vi "Multiple TransducersNathanOnboardClock.vi"() -> ()   [LabVIEW 2015]
doc: "Reads force and torque values from multiple ATI transducers."
uses:
  <vilib>/DAQmx/read.llb/DAQmx Read (Analog 2D DBL NChan NSamp).vi
  <vilib>/Analysis/baseanly.llb/A x Vector.vi
  <vilib>/DAQmx/create/channels.llb/DAQmx Create Channel (AI-Voltage-Basic).vi
  <vilib>/DAQmx/configure/timing.llb/DAQmx Timing (Sample Clock).vi
  <vilib>/DAQmx/configure/trigger.llb/DAQmx Start Trigger (Digital Edge).vi
  <vilib>/DAQmx/miscellaneous.llb/DAQmx Fill In Error Info.vi
  <vilib>/Analysis/NI_AALBase.lvlib
panel:
  in  "User Torque Units":string
  in  "User Force Units":string
  in  "Calibration Units":T1(array[cluster])
  in  "Tool Transforms":T2(array[cluster])
  in  "Scan Lists":string[](array[string])=["dev1/ai0:5,dev1/ai6:11"]
  in  "Enable Transducer":bool[](array[boolean])
  in  "Filename":path
  in  "Connection Mode":i32(ring)=-1 items=["default"=-1, "RSE"=10083, "NRSE"=10078, "Differential"=10106, "Pseudodifferential"=12529]
  in  "Bias All":bool
  in  "Start Saving Data":bool
  in  "Bias Transducer":bool[](array[boolean])
  in  "Append Data?":bool
  in  "Samples to Read at a time":i32=50
  out "Voltages":dbl[][](array[numeric])
  in  "Buffer Size":i32=1000
  in  "Sample Rate":dbl=1000.0
  out "F/T Values":dbl[][][](array[numeric])
  in  "Calibration Files":path[](array[path])=[path "C:/Program Files/ATI DAQ FT/FT5816.cal", path "C:/Program Files/ATI DAQ FT/FT5395.cal"]
  # "For assistance, turn on context help and examine\nthe help text for each control."
  # "Fx"
  # "Fy"
  # "Fz"
  # "Tx"
  # "Ty"
  # "Tz"
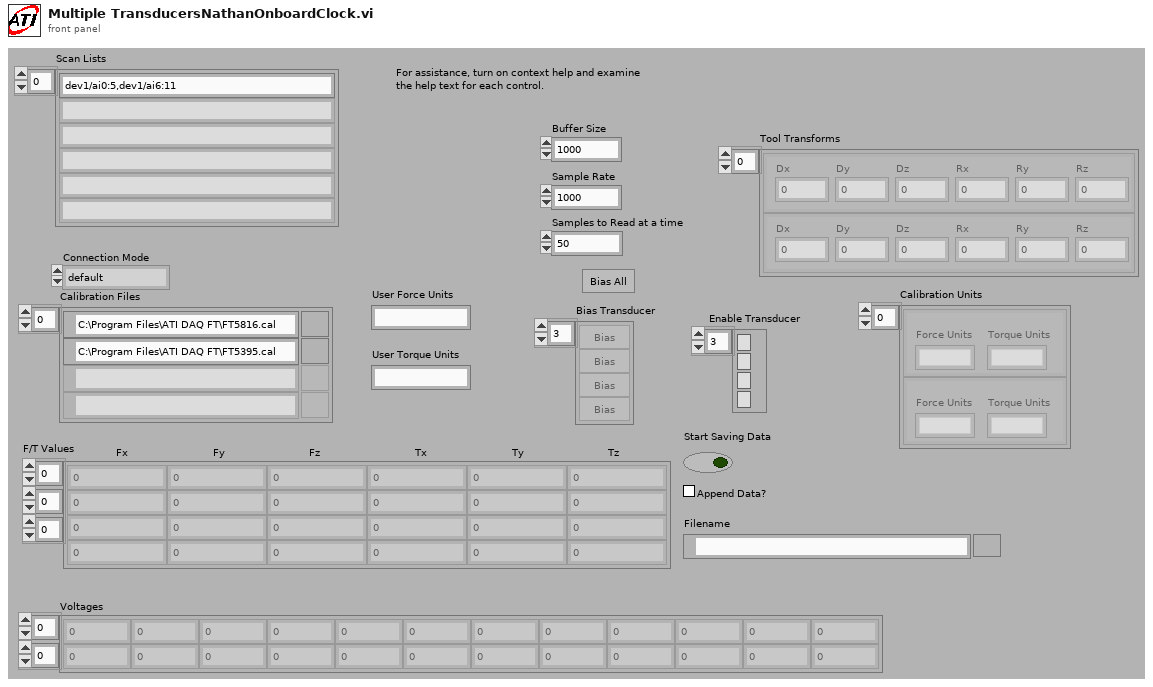
[diagram p1: front panel]
types:
  T1 = cluster{"Force Units":string, "Torque Units":string}[]
  T2 = cluster{"Dx":dbl, "Dy":dbl, "Dz":dbl, "Rx":dbl, "Ry":dbl, "Rz":dbl}[]
  T3 = cluster{"Calibration Force Units":string, "Calibration Torque Units":string}
  T4 = enum16{"open", "open or create", "create or replace", "create", "open (read only)"}
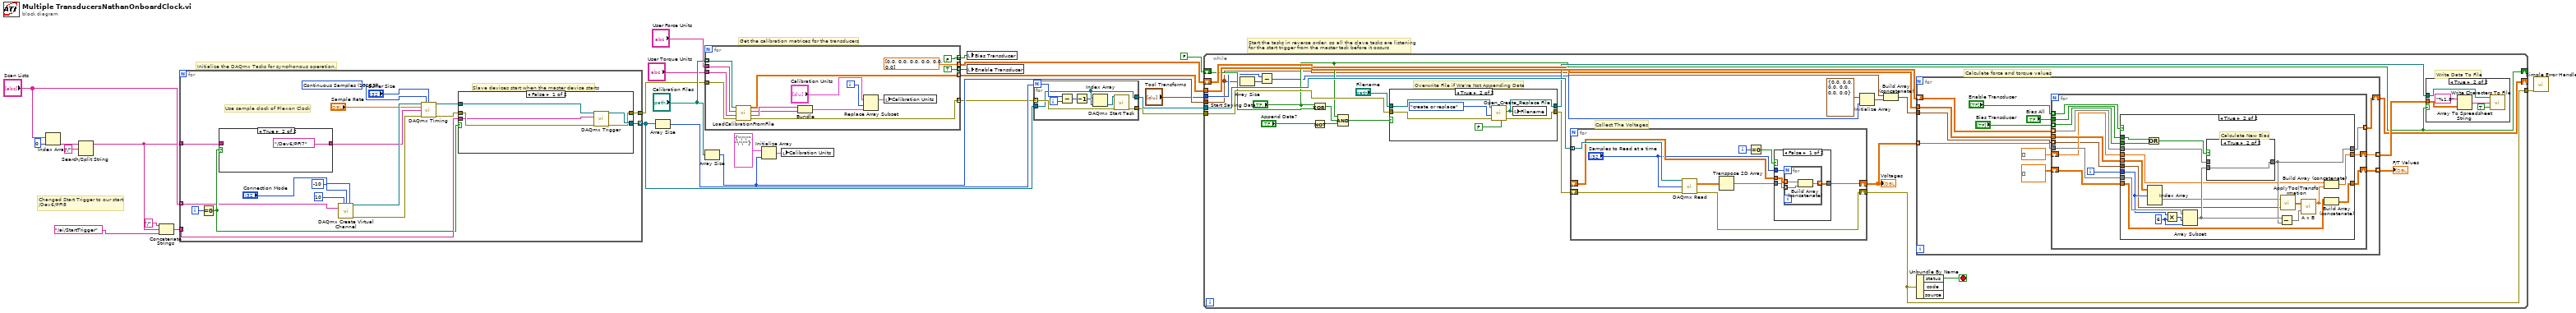
[diagram p0: block diagram]
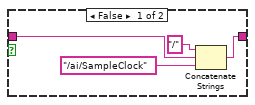
[diagram p7: hidden frame]
diagram:
  # "Changed Start Trigger to our start\n/Dev6/PFI8"
  # "Initialize the DAQmx Tasks for syncrhonous operation."
  # "Get the calibration matrices for the transducers"
  # "Start the tasks in reverse order, so all the slave tasks are listening \nfor the start trigger from the master task before it occurs"
  n1 = Index Array(array="Scan Lists", index=0) -> (element=w15:string)
  n2 = Search/Split String(string=w15, search string/char (-)="/") -> (substring before match=w13:string)  [unwired: 1 in, 2 out]
  n3 = Concatenate Strings("/", w13, "/ai/StartTrigger") -> (w27:string)
  n4 = for {
    tunnel: w27 -> [w39]
    tunnel: [w36] -> w3
    tunnel: [w30] -> w18 mode=indexing
    tunnel: "Scan Lists" -> [w29] mode=indexing
    tunnel: w13 -> [w28]
    i -> [w41]
    w43 = 10123 items=["Finite Samples"=10178, "Continuous Samples"=10123, "Hardware Timed Single Point"=12522] ("sample mode")
    # "Slave devices start when the master device starts"
    # "Use sample clock of Plexon Clock"
    n5 = Equal To 0?(x=w41) -> (x = 0?=w35:bool)
    n6 = case shown="True" w35 {
      tunnel: [w47 tag "/Dev6/PFI7"] -> w34
      tunnel: w28 -> [w46 _]
      frame False {
        n7 = Concatenate Strings("/", w46, "/ai/SampleClock") -> (w47:string)
      }
      frame True {
      }
    }
    n8 = call-poly <vilib>:"DAQmx Create Virtual Channel.vi"("maximum value"=10, "minimum value"=-10, "input terminal configuration"="Connection Mode", "physical channels"=w29) -> ("task out"=w45:refnum<k21>, "error out"=w38:errorcluster)  [unwired: 10 in]
    n9 = call-poly <vilib>:"DAQmx Timing.vi"("task/channels in"=w45, "sample mode"=w43, "samples per channel"="Buffer Size", "rate"="Sample Rate", "source"=w34, "error in"=w38) -> ("task out"=w40:refnum<k21>, "error out"=w37:errorcluster)  [unwired: 8 in]
    n10 = case shown="False" w35 {
      tunnel: w40 -> [w55 w57]
      tunnel: [w54 w57] -> w30
      tunnel: w39 -> [w51 _]
      tunnel: w37 -> [w53 w56]
      tunnel: [w52 w56] -> w36
      frame False {
        n11 = call-poly <vilib>:"DAQmx Trigger.vi"("task/channels in"=w55, "source"=w51, "error in"=w53) -> ("task out"=w54:refnum<k21>, "error out"=w52:errorcluster)  [unwired: 11 in]
      }
      frame True {
      }
    }
  }
  n12 = Array Size(array=w18) -> (size(s)=w20:i32)
  n13 = for {
    tunnel: "Calibration Files" -> [w70] mode=indexing
    tunnel: [FALSE] -> w24 mode=indexing
    tunnel: [TRUE] -> w22 mode=indexing
    tunnel: [w68] -> w21 mode=indexing
    tunnel: [dbl[] [0.0, 0.0, 0.0, 0.0, 0.0, 0.0]] -> w11 mode=indexing
    tunnel: "User Force Units" -> [w61]
    tunnel: "User Torque Units" -> [w60]
    tunnel: w3 -> [w59]
    tunnel: [w58] -> w2 mode=indexing
    i -> [w67]
    n14 = call "LoadCalibrationFromFile.vi"("Error In"=w59, "User Torque Units"=w60, "User Force Units"=w61, "Cal File Path"=w70) -> ("Error Out"=w58:errorcluster, "Calibration Force Units"=w64:string, "Calibration Torque Units"=w63:string, "Calibration Matrix"=w68:dbl[][])
    n15 = Bundle("Calibration Force Units"=w64, "Calibration Torque Units"=w63) -> (w65:T3)  [unwired: 1 in]
    n16 = Replace Array Subset(array="Calibration Units", new element=w65, index=w67) -> (w62:T1)
    n17 = local write "Calibration Units"(w62) -> ()
  }
  n18 = Array Size(array="Calibration Files") -> (size(s)=w7:i32)
  n19 = Initialize Array(cluster{string, string} {"\"\"", "\"\""}, w7) -> (w6:cluster{string, string}[])
  n20 = local write "Calibration Units"(w6) -> ()
  n21 = local write "Bias Transducer"(w24) -> ()
  n22 = local write "Enable Transducer"(w22) -> ()
  n23 = for {
    N: w20 -> [w80]
    tunnel: w18 -> [w75]
    tunnel: w2 -> [w76] mode=indexing
    tunnel: [w75] -> w26
    tunnel: [w73] -> w12
    i -> [w79]
    n24 = Subtract(x=w80, y=w79) -> (x-y=w78:i32)
    n25 = Decrement(x=w78) -> (x-1=w74:i32)
    n26 = Index Array(array=w75, index=w74) -> (element=w77:refnum<k21>)
    n27 = call <vilib>:"DAQmx Start Task.vi"("task/channels in"=w77, "error in"=w76) -> ("error out"=w73:errorcluster)  [unwired: 12 in, 1 out]
  }
  n28 = while {
    tunnel: w26 -> [w106]
    tunnel: w21 -> [w104]
    shift-right: [w93] -> _
    shift-left: w11 -> [w102]
    shift-right: ["Start Saving Data"] -> _
    shift-left: FALSE -> [w92]
    tunnel: w12 -> [w96]
    tunnel: [w88] -> w19
    tunnel: "Tool Transforms" -> [w83]
    tunnel: w7 -> [w86]
    stop <- w89 stop-if-true
    # "Write Data To File"
    # "Overwrite File if We're Not Appending Data"
    # "Calculate force and torque values"
    # "Collect The Voltages"
    n29 = Array Size(array=w83) -> (size(s)=w85:i32)
    n30 = Subtract(x=w86, y=w85) -> (x-y=w84:i32)
    n31 = Exclusive Or(1:w92, 2:"Start Saving Data") -> (0:w91:bool)
    n32 = Not(x="Append Data?") -> (.not. x?=w98:bool)
    n33 = Compound Arithmetic op=AND("Start Saving Data", w91, w98) -> (w101:bool)
    n34 = case shown="True" w101 {
      tunnel: "Filename" -> [w113 w119]
      tunnel: [w113 w114] -> w97
      tunnel: w96 -> [w112 w118]
      tunnel: [w112 w117] -> w95
      frame False {
      }
      frame True {
        n35 = call <vilib>:"Open_Create_Replace File.vi"("advisory dialog? (display:T)"=FALSE, "error in (no error)"=w118, "function (open:0)"=T4."create or replace", "file path"=w119) -> ("error out"=w117:errorcluster, "new file path"=w114:path)  [unwired: 4 in, 2 out]
        n36 = local write "Filename"(w114) -> ()
      }
    }
    n37 = for {
      tunnel: w106 -> [w179] mode=indexing
      shift-right: [w176] -> w88
      shift-left: w95 -> [w178]
      shift-right: [w173] -> w105
      shift-left: _ -> [w171]
      i -> [w175]
      n38 = call-poly <vilib>:"DAQmx Read.vi"("task/channels in"=w179, "number of samples per channel"="Samples to Read at a time", "error in"=w178) -> ("data"=w177:dbl[][], "error out"=w176:errorcluster)  [unwired: 10 in, 1 out]
      n39 = Transpose 2D Array(2D array=w177) -> (transposed array=w172:dbl[][])
      n40 = Equal To 0?(x=w175) -> (x = 0?=w174:bool)
      n41 = case shown="False" w174 {
        tunnel: [w181 w187] -> w173
        tunnel: w172 -> [w182 w187]
        tunnel: w171 -> [w183 _]
        tunnel: "Samples to Read at a time" -> [w180 _]
        frame False {
          n42 = for {
            N: w180 -> [_]
            tunnel: w183 -> [w186] mode=indexing
            tunnel: w182 -> [w185] mode=indexing
            tunnel: [w184] -> w181 mode=indexing
            n43 = Build Array (concatenate)(w186, w185) -> (w184:dbl[])
          }
        }
        frame True {
        }
      }
    }
    "Voltages" <- w105
    n44 = Initialize Array(cluster{dbl, dbl, dbl, dbl, dbl, dbl} {0.0, 0.0, 0.0, 0.0, 0.0, 0.0}, w84) -> (w82:cluster{dbl, dbl, dbl, dbl, dbl, dbl}[])
    n45 = Build Array (concatenate)(w83, w82) -> (w81:T2)
    n46 = for {
      tunnel: w105 -> [w130] mode=indexing
      tunnel: w104 -> [w131]
      tunnel: [w121] -> w103 mode=indexing
      tunnel: [w126] -> w94 mode=indexing
      shift-right: [w124] -> w93
      shift-left: w102 -> [w129]
      tunnel: w81 -> [w120]
      n47 = for {
        tunnel: w131 -> [w139]
        tunnel: w130 -> [w144]
        tunnel: w129 -> [w142] mode=indexing
        tunnel: "Bias Transducer" -> [w143] mode=indexing
        tunnel: [w141] -> w124 mode=indexing
        shift-right: [w136] -> w126
        shift-left: dbl[] [] -> [w137]
        tunnel: "Bias All" -> [w140]
        tunnel: "Enable Transducer" -> [w135] mode=indexing
        shift-right: [w133] -> w121
        shift-left: sgl[][] [] -> [w134]
        tunnel: w120 -> [w132] mode=indexing
        i -> [w138]
        n48 = case shown="True" w135 {
          tunnel: w144 -> [_ w165]
          tunnel: w143 -> [_ w164]
          tunnel: w142 -> [w147 w162]
          tunnel: [w147 w160] -> w141
          tunnel: w140 -> [_ w158]
          tunnel: w139 -> [_ w157]
          tunnel: w138 -> [_ w156]
          tunnel: w137 -> [w146 w155]
          tunnel: [w146 w154] -> w136
          tunnel: w134 -> [w145 w153]
          tunnel: [w145 w151] -> w133
          tunnel: w132 -> [_ w149]
          frame False {
          }
          frame True {
            w166 = 6
            # "Calculate New Bias"
            n49 = Or(x=w158, y=w164) -> (x .or. y?=w163:bool)
            n50 = Index Array(array=w157, index (dim 0)=w156) -> (element=w150:dbl[][])  [unwired: 2 in]
            n51 = Multiply(x=w156, y=w166) -> (x*y=w167:i32)
            n52 = Array Subset(array=w165, index=w167, length=w166) -> (w161:dbl[])
            n53 = case shown="True" w163 {
              tunnel: w161 -> [_ w169]
              tunnel: [w168 w169] -> w160
              tunnel: w162 -> [w168 _]
              frame False {
              }
              frame True {
              }
            }
            n54 = Subtract(x=w161, y=w160) -> (x-y=w159:dbl[])
            n55 = call "ApplyToolTransformation.vi"("Transform"=w149, "Calibration Matrix"=w150) -> ("Transformed Calibration Matrix"=w148:dbl[][])
            n56 = call-poly <vilib>:"A x B.vi"("Vector"=w159, "A"=w148) -> ("A x Vector"=w152:dbl[])  [unwired: 1 out]
            n57 = Build Array (concatenate)(w155, w152) -> (w154:dbl[])
            n58 = Build Array (concatenate)(w153, w152) -> (w151:dbl[][])
          }
        }
      }
    }
    "F/T Values" <- w103
    n59 = Unbundle By Name(w88) -> ("status"=w89:bool)  [unwired: 2 out]
    n60 = case shown="True" "Start Saving Data" {
      tunnel: w97 -> [_ w111]
      tunnel: w94 -> [_ w108]
      frame False {
      }
      frame True {
        n61 = Array To Spreadsheet String(array=w108, 3:"%1.8" ("format string")) -> (spreadsheet string=w107:string)  [unwired: 1 in]
        n62 = call <vilib>:"Write Characters To File.vi"("append to file? (new file:F)"=TRUE, "character string"=w107, "file path (dialog if empty)"=w111) -> ()  [unwired: 2 in, 1 out]
      }
    }
  }
  n63 = call <vilib>:"Simple Error Handler.vi"("error in (no error)"=w19) -> ()  [unwired: 4 in, 5 out]
